vi "channel operation tests.vi"() -> ()   [LabVIEW 2013, in "sample module tests.lvlib"]
uses:
  sample module tests.lvlib
  channel/channel classification.ctl
  module/configuration/sample module configuration.lvclass
  channel/TBM channel.lvclass
  root configuration/TBM configuration.lvclass
panel:
  out "channels match":bool
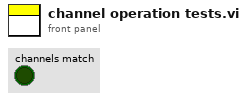
[diagram p1: front panel]
types:
  T1 = typedef "TBM channel.lvclass/channel classification.ctl" = enum16{"input data", "output data", "processing parameter", "processing result"}
  T2 = typedef "tag bus.lvlib/tag descriptor.lvclass/Data Type.ctl" = enum16{"Double", "Single", "I64", "I32", "I16", "I8", "U64", "U32", "U16", "U8", "Boolean", "String", "Array of Double", "Array of Single", "Array of I64", "Array of I32", "Array of I16", "Array of I8", "Array of U64", "Array of U32", "Array of U16", "Array of U8", "Array of Boolean", "Array of String"}
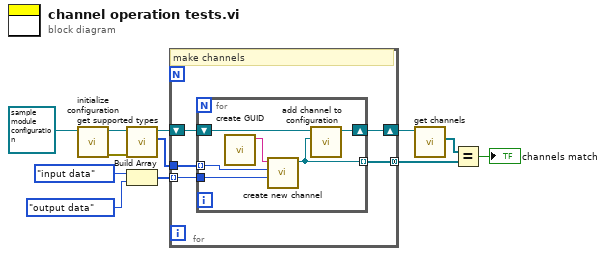
[diagram p0: block diagram]
diagram:
  n1 = call-dynamic "initialize configuration.vi"("configuration in"=refnum<class "sample module configuration.lvclass"> refnum ("sample module configuration")) -> ("error out"=w4:errorcluster, "configuration out"=w5:refnum<class "sample module configuration.lvclass">)  [unwired: 8 in, 1 out]
  n2 = call-dynamic "get supported types.vi"("error in"=w4, "sample module configuration in"=w5) -> ("supported types"=w3:T2[], "sample module configuration out"=w2:refnum<class "sample module configuration.lvclass">)  [unwired: 7 in, 1 out]
  n3 = Build Array(channel_classification."input data" ("channel classification"), channel_classification."output data" ("channel classification")) -> (w10:T1[])
  n4 = for {
    tunnel: w10 -> [w17] mode=indexing
    tunnel: [w15] -> w7 mode=concatenating
    tunnel: w3 -> [w16]
    shift-right: [w13] -> w1
    shift-left: w2 -> [w14]
    # "make channels"
    n5 = for {
      tunnel: w17 -> [w23]
      tunnel: [w18] -> w15 mode=indexing
      tunnel: w16 -> [w22] mode=indexing
      shift-right: [w19] -> w13
      shift-left: w14 -> [w20]
      n6 = call "create GUID.vi"() -> ("uuid"=w21:string)  [unwired: 11 in]
      n7 = call "create new channel.vi"("channel classification"=w23, "data type"=w22, "channel name"=w21) -> ("channel"=w18:refnum<class "TBM channel.lvclass">)  [unwired: 8 in]
      n8 = call "add channel to configuration.vi"("channel"=w18, "sample module configuration in"=w20) -> ("sample module configuration out"=w19:refnum<class "sample module configuration.lvclass">)  [unwired: 8 in, 1 out]
    }
  }
  n9 = call-dynamic "get channels.vi"("module configuration in"=w1) -> ("channels"=w9:refnum<class "TBM channel.lvclass">[])  [unwired: 9 in, 1 out]
  n10 = Equal?(x=w9, y=w7) -> (x = y?=→"channels match":bool)
